vi "Generate Unique Header.vi"(8 "error in":errorcluster, 11 "Alicat Data in":refnum<class "Alicat Data.lvclass">) -> (0 "error out":errorcluster, 2 "Header":string[](array[string]), 3 "Alicat Data out":refnum<class "Alicat Data.lvclass">)   [LabVIEW 2015, in "Alicat Lib.lvlib" / "Alicat Data.lvclass"]
uses:
  Alicat Data.lvclass
  <vilib>/MSR Consulting, LLC/General Reuse/Data/Data.lvclass/Data.ctl
  <vilib>/MSR Consulting, LLC/General Reuse/Data/Read Data ID.vi
  <vilib>/MSR Consulting, LLC/General Reuse/Data/Data.lvclass
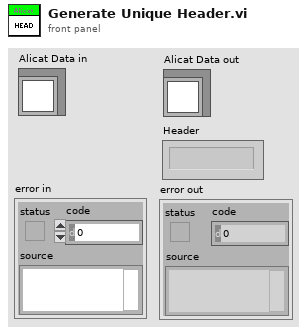
[diagram p1: front panel]
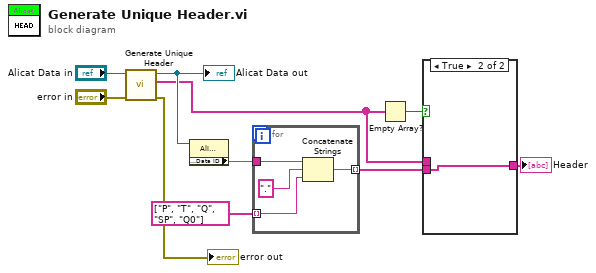
[diagram p0: block diagram]
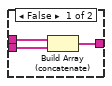
[diagram p2: hidden frame]
diagram:
  n1 = call-parent "Generate Unique Header.vi"("error in"="error in", "Data in"="Alicat Data in") -> ("error out"=→"error out":errorcluster, "Header"=w2:string[], "Data out"=w6:refnum<class "Alicat Data.lvclass">)  [unwired: 7 in]
  "Alicat Data out" <- w6
  n2 = property class="Alicat Data"(reference=w6) -> ("Accessors:Data ID"=w5:string)  [unwired: 1 in, 2 out]
  n3 = for {
    tunnel: string[] ["P", "T", "Q", "SP", "Q0"] -> [w11] mode=indexing
    tunnel: w5 -> [w14]
    tunnel: [w13] -> w4 mode=indexing
    n4 = Concatenate Strings(w14, "." ("string"), w11) -> (w13:string)
  }
  n5 = Empty Array?(array=w2) -> (empty?=w1:bool)
  n6 = case shown="True" w1 {
    tunnel: w4 -> [w17 w18]
    tunnel: w2 -> [w16 _]
    tunnel: [w15 w18] -> w3
    frame False {
      n7 = Build Array (concatenate)(w16, w17) -> (w15:string[])
    }
    frame True {
    }
  }
  "Header" <- w3
